vi "FVIR_LDO_Alicat_GasMeter.vi"(8 "error in":errorcluster, 10 "VISA Refnum in":refnum<visa-resource-name>="ALICAT_100SLPM", 11 "Message Queues":T1) -> (0 "error out":errorcluster)   [LabVIEW 2020]
uses:
  Message Queue/All Message Queues.ctl
  Message Queue/Message Cluster.ctl
  Modbus/Modbus Gas Meter Data.ctl
  Drivers/Alicat LabVIEW Drivers 2v1/Sub-VIs/Data Cluster.ctl
  Drivers/Alicat LabVIEW Drivers 2v1/Sub-VIs/Units of Measure.ctl
  Message Queue/Enqueue Message (Single).vi
  Message Queue/Message Queue.lvlib
panel:
  in  "Debug":bool
  out "Debug":string[](array[string])
  out "Loop Count":i32
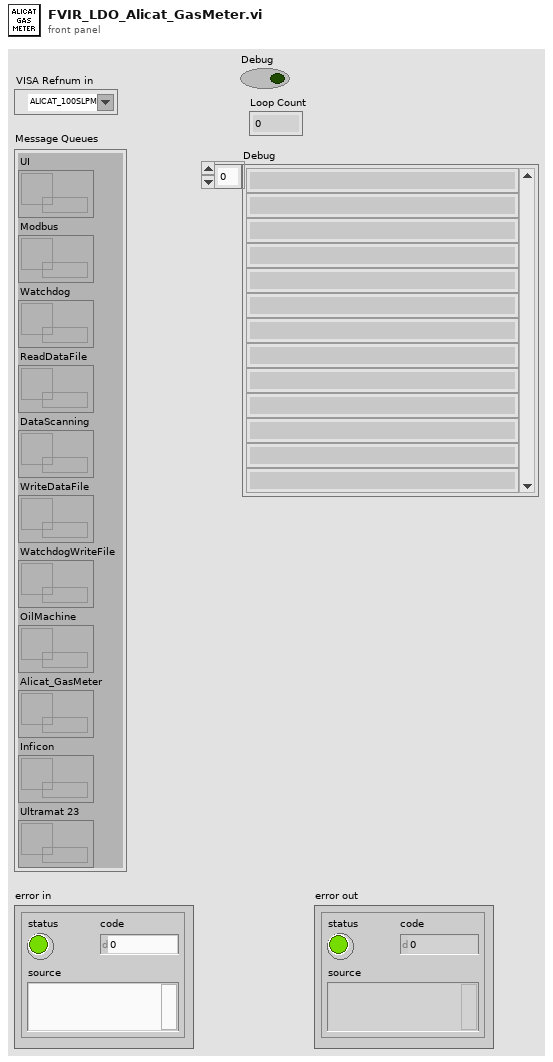
[diagram p1: front panel]
types:
  T1 = typedef "Message Queue.lvlib/All Message Queues.ctl" = cluster{"UI":refnum<queue>, "Modbus":refnum<queue>, "Watchdog":refnum<queue>, "ReadDataFile":refnum<queue>, "DataScanning":refnum<queue>, "WriteDataFile":refnum<queue>, "WatchdogWriteFile":refnum<queue>, "OilMachine":refnum<queue>, "Alicat_GasMeter":refnum<queue>, "Inficon":refnum<queue>, "Ultramat 23":refnum<queue>}
  T2 = cluster{"Absolute Press.":bool, "Gauge/Diff. Press.":bool, "Barometric Press.":bool, "Temperature":bool, "Volumetric":bool, "Mass Flow":bool, "Setpoint":bool, "Valve Drive":bool, "Totalizer":bool, "Tot. Timer [s]":bool, "Tot. Avg. Flow":bool, "Tot. Peak Flow":bool, "Gas Selected":bool, "Log Data":bool}
  T3 = typedef "Modbus Gas Meter Data.ctl" = cluster{"Data Cluster":T4, "Units of Measure Input":T5, "Header Array":string[]}
  T4 = typedef "Data Cluster.ctl" = cluster{"Absolute Pressure":dbl, "Gauge/Diff. Pressure":dbl, "Barometric Pressure":dbl, "Temperature":dbl, "Volumetric Flow":dbl, "Mass Flow":dbl, "Setpoint":dbl, "Valve Drive":dbl, "Totalizer":dbl, "[hr]":dbl, "[min]":dbl, "[sec]":dbl, "Totalizer Average Flow":dbl, "Totalizer Peak Flow":dbl, "Gas selected":string}
  T5 = typedef "Units of Measure.ctl" = cluster{"Abs. Pressure":string, "Gauge/Diff. Press.":string, "Barometric Press.":string, "Temperature":string, "Volume":string, "Mass":string, "Setpoint":string, "Valve Drive":string, "Totalizer":string, "Tot. Timer":string, "Tot. Avg. Flow":string, "Tot. Peak Flow":string}
  T6 = typedef "Data Frame.ctl" = cluster{"Absolute Pressure":bool, "Gauge/Diff. Pressure":bool, "Barometric Pressure":bool, "Temperature":bool, "Volumetric":bool, "Mass":bool, "Setpoint":bool, "Valve Drive":bool, "Totalizer":bool, "Totalizer Timer":bool, "Totalizer Average Flow":bool, "Totalizer Peak Flow":bool, "Gas Selected":bool, "Tot. Timer Format":u16}
  T7 = typedef "FMA1600A Units String.ctl" = cluster{"Software Rev":string, "Model Number":string, "Manufacturer Info":string, "Software Sub-Rev":string, "Board Rev":string, "Units of Measure Input":T5}
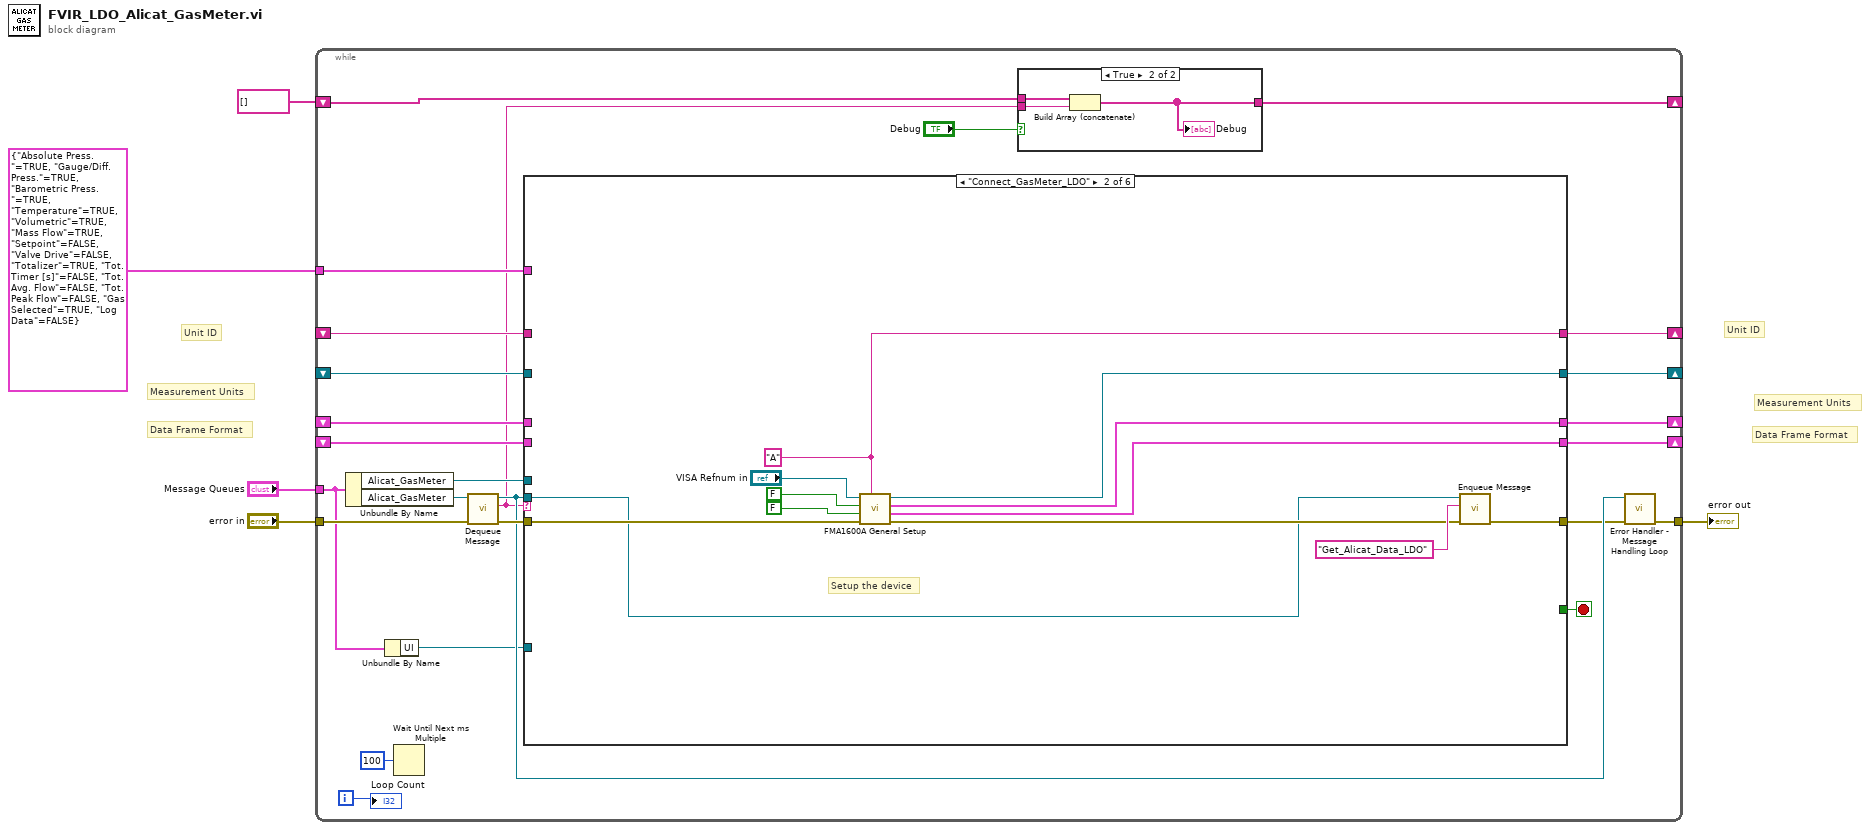
[diagram p0: block diagram]
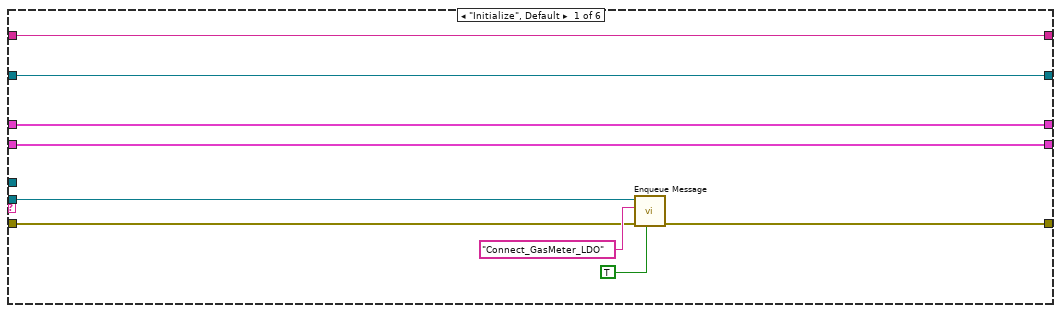
[diagram p3: hidden frame]
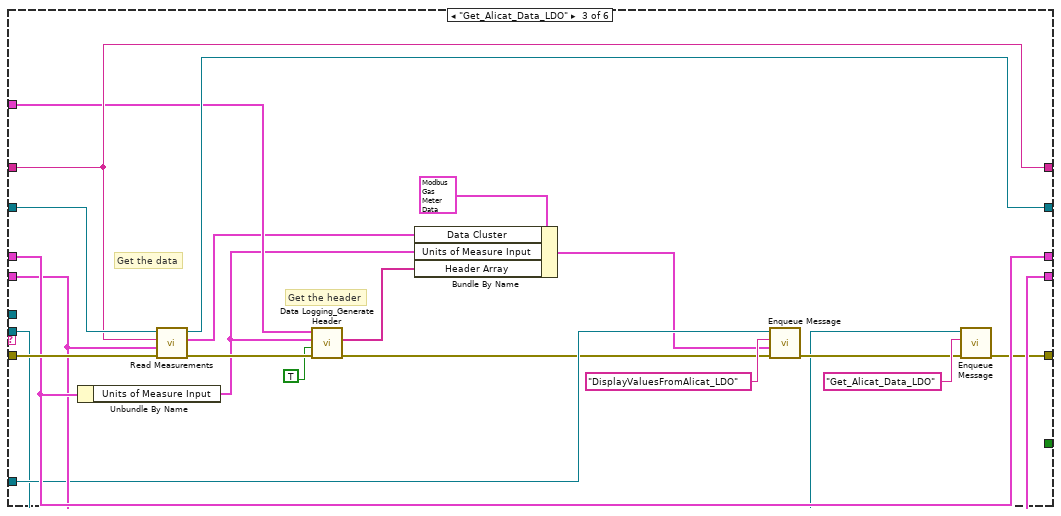
[diagram p4: hidden frame]
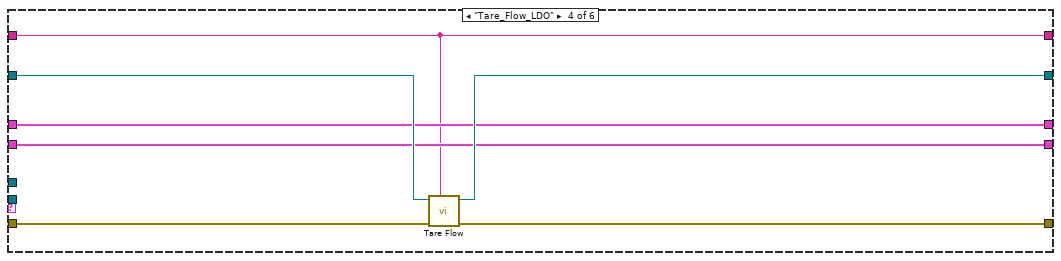
[diagram p5: hidden frame]
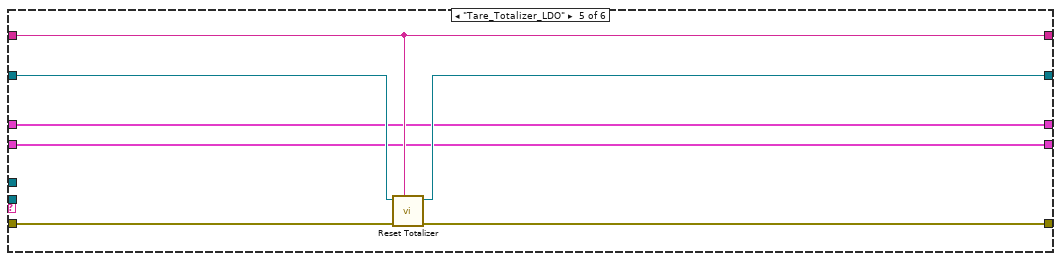
[diagram p6: hidden frame]
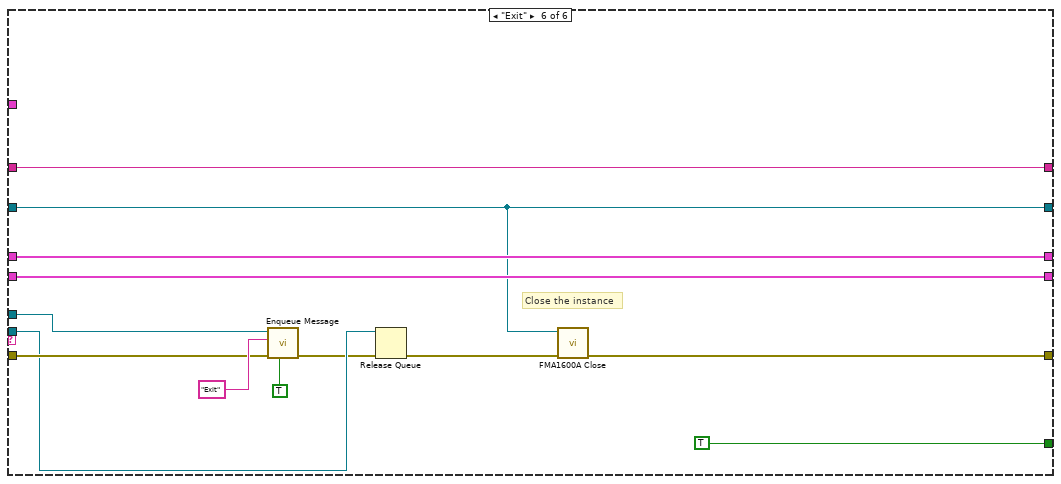
[diagram p7: hidden frame]
diagram:
  # "Unit ID"
  # "Data Frame Format"
  # "Measurement Units"
  # "Unit ID"
  # "Data Frame Format"
  # "Measurement Units"
  n1 = while {
    tunnel: "Message Queues" -> [w11]
    tunnel: "error in" -> [w29]
    tunnel: [w24] -> w3
    shift-right: [w22] -> _
    shift-left: _ -> [w21]
    shift-right: [w18] -> _
    shift-left: _ -> [w15]
    shift-right: [w17] -> _
    shift-left: _ -> [w16]
    shift-right: [w14] -> _
    shift-left: _ -> [w13]
    tunnel: T2 {"Absolute Press."=TRUE, "Gauge/Diff. Press."=TRUE, "Barometric Press."=TRUE, "Temperature"=TRUE, "Volumetric"=TRUE, "Mass Flow"=TRUE, "Setpoint"=FALSE, "Valve Drive"=FALSE, "Totalizer"=TRUE, "Tot. Timer [s]"=FALSE, "Tot. Avg. Flow"=FALSE, "Tot. Peak Flow"=FALSE, "Gas Selected"=TRUE, "Log Data"=FALSE} ("Data Logging Options") -> [w12]
    shift-right: [w7] -> _
    shift-left: string[] [] -> [w8]
    i -> [w19]
    stop <- w27 stop-if-true
    n2 = Unbundle By Name(w11) -> ("Alicat_GasMeter"=w26:refnum<queue>, "Alicat_GasMeter"=w30:refnum<queue>)
    n3 = Unbundle By Name(w11) -> ("UI"=w10:refnum<queue>)
    n4 = Wait Until Next ms Multiple(millisecond multiple=u32 100) -> ()  [unwired: 1 out]
    n5 = call "Dequeue Message.vi"("error in (no error)"=w29, "Message Queue"=w30) -> ("error out"=w28:errorcluster, "Message"=w9:string, "dup Message Queue"=w25:refnum<queue>)  [unwired: 6 in, 1 out]
    n6 = case shown="\"Connect_GasMeter_LDO\"" w9 {
      tunnel: w28 -> [w38 w52 w73 w83 w90 w99]
      tunnel: [w37 w45 w63 w82 w89 w95] -> w23
      tunnel: [_ _ _ _ _ TRUE] -> w27
      tunnel: w26 -> [_ _ _ _ _ w100]
      tunnel: w25 -> [w36 w44 w62 _ _ w98]
      tunnel: [w43 w51 w74 w80 w86 w91] -> w22
      tunnel: w21 -> [w43 _ w72 w81 w88 w91]
      tunnel: [w41 w50 w70 w79 w85 w93] -> w18
      tunnel: [w40 w49 w69 w78 w84 w92] -> w17
      tunnel: w16 -> [w40 _ w69 w78 w84 w92]
      tunnel: w15 -> [w41 _ w70 w79 w85 w93]
      tunnel: [w42 w48 w71 w77 w87 w94] -> w14
      tunnel: w13 -> [w42 _ w71 w77 w87 w94]
      tunnel: w12 -> [_ _ w68 _ _ _]
      tunnel: w10 -> [_ _ w66 _ _ _]
      frame "Initialize", Default {
        n7 = call-poly "Enqueue Message.vi"("Priority Message? (F)"=TRUE, "error in (no error)"=w38, "Message"="Connect_GasMeter_LDO", "Message Queue"=w36) -> ("error out"=w37:errorcluster)  [unwired: 6 in, 1 out]
      }
      frame "Connect_GasMeter_LDO" {
        w48 = "A" ("Unit ID")
        # "Setup the device"
        n8 = call "FMA1600A General Setup.vi"("Unit ID"=w48, "error in (no error)"=w52, "Select Gas?"=FALSE, "Set STP Register"=FALSE, "VISA Refnum in"="VISA Refnum in") -> ("error out"=w46:errorcluster, "Data Frame Format"=w49:T6, "Measurement Units"=w50:T7, "VISA Refnum out"=w51:refnum<visa-resource-name>)  [unwired: 3 in]
        n9 = call-poly "Enqueue Message.vi"("error in (no error)"=w46, "Message"="Get_Alicat_Data_LDO", "Message Queue"=w44) -> ("error out"=w45:errorcluster)  [unwired: 7 in, 1 out]
      }
      frame "Get_Alicat_Data_LDO" {
        # "Get the header"
        # "Get the data"
        n10 = Unbundle By Name(w70) -> ("Units of Measure Input"=w58:T5)
        n11 = call "Read Measurements.vi"("error in"=w73, "Data Frame Format In"=w69, "Unit ID (A)"=w71, "VISA Session In"=w72) -> ("error out"=w76:errorcluster, "Data Cluster"=w59:T4, "VISA Session Out"=w74:refnum<visa-resource-name>)  [unwired: 5 out]
        n12 = call "Data Logging_Generate Header.vi"("error in"=w76, "Include Units\nin Header (F)"=TRUE ("Include Units\nin Header (default is F)"), "Units of Measure Input"=w58, "Data Logging Options"=w68) -> ("error out"=w61:errorcluster, "Header Array"=w57:string[])  [unwired: 5 in, 1 out]
        n13 = Bundle By Name(cluster=T3 {"Data Cluster"={"Absolute Pressure"=0.0, "Gauge/Diff. Pressure"=0.0, "Barometric Pressure"=0.0, "Temperature"=0.0, "Volumetric Flow"=0.0, "Mass Flow"=0.0, "Setpoint"=0.0, "Valve Drive"=0.0, "Totalizer"=0.0, "[hr]"=0.0, "[min]"=0.0, "[sec]"=0.0, "Totalizer Average Flow"=0.0, "Totalizer Peak Flow"=0.0, "Gas selected"=""}, "Units of Measure Input"={"Abs. Pressure"="", "Gauge/Diff. Press."="", "Barometric Press."="", "Temperature"="", "Volume"="", "Mass"="", "Setpoint"="", "Valve Drive"="", "Totalizer"="", "Tot. Timer"="", "Tot. Avg. Flow"="", "Tot. Peak Flow"=""}, "Header Array"=[]} ("Gas Data"), "Data Cluster"=w59, "Units of Measure Input"=w58, "Header Array"=w57) -> (w56:T3)
        n14 = call-poly "Enqueue Message.vi"("error in (no error)"=w61, "Message Data"=w56, "Message"="DisplayValuesFromAlicat_LDO", "Message Queue"=w66) -> ("error out"=w64:errorcluster)  [unwired: 6 in, 1 out]
        n15 = call-poly "Enqueue Message.vi"("error in (no error)"=w64, "Message"="Get_Alicat_Data_LDO", "Message Queue"=w62) -> ("error out"=w63:errorcluster)  [unwired: 7 in, 1 out]
      }
      frame "Tare_Flow_LDO" {
        n16 = call "Tare Flow.vi"("Unit ID (A)"=w77, "error in"=w83, "VISA Session In"=w81) -> ("error out"=w82:errorcluster, "VISA Session Out"=w80:refnum<visa-resource-name>)  [unwired: 7 in]
      }
      frame "Tare_Totalizer_LDO" {
        n17 = call "Reset Totalizer.vi"("Unit ID (A)"=w87, "error in"=w90, "VISA Session In"=w88) -> ("error out"=w89:errorcluster, "VISA Session Out"=w86:refnum<visa-resource-name>)  [unwired: 6 in, 1 out]
      }
      frame "Exit" {
        # "Close the instance"
        n18 = call-poly "Enqueue Message.vi"("Priority Message? (F)"=TRUE, "error in (no error)"=w99, "Message"="Exit", "Message Queue"=w100) -> ("error out"=w97:errorcluster)  [unwired: 6 in, 1 out]
        n19 = Release Queue(queue=w98, error in (no error)=w97) -> (error out=w96:errorcluster)  [unwired: 1 in, 2 out]
        n20 = call "FMA1600A Close.vi"("error in (no error)"=w96, "VISA Refnum in"=w91) -> ("error out"=w95:errorcluster)  [unwired: 9 in]
      }
    }
    n21 = case shown="True" "Debug" {
      tunnel: w9 -> [_ w34]
      tunnel: w8 -> [w31 w33]
      tunnel: [w31 w32] -> w7
      frame False {
      }
      frame True {
        n22 = Build Array (concatenate)(w33, w34) -> (w32:string[])
        "Debug" <- w32
      }
    }
    n23 = call "Error Handler - Message Handling Loop.vi"("error in (no error)"=w23, "Message Queue"=w25) -> ("dup error in"=w24:errorcluster)  [unwired: 8 in, 1 out]
    "Loop Count" <- w19
  }
  "error out" <- w3
